vi "TDMS Advanced Asynchronous Write Speed Test.vi"() -> ()   [LabVIEW 2023]
doc: "This example demonstrates how to benchmark the streaming performance when you use the TDMS Advanced Asynchronous File I/O functions to write data to a .tdms file. This VI measures the time it takes to continuously write data from system memory to a .tdms file on the hard disk or a RAID array. This VI then calculates the average data throughput in bytes/second."
uses:
  <vilib>/Utility/tdmsutil.llb/TDMS Generate Random Data (I16).vi
panel:
  in  "Disable Buffering? (T)":bool=TRUE
  out "Bytes/second":dbl format="%#_4p"
  in  "Max Asynchronous Writes (4)":u32=4 step=1
  out "Current Number of Writes":i32
  out "Total Number of Writes":u64
  in  "Total Bytes to Write":u64=419430400
  in  "Write Block Size (bytes)":u64=4194304 step=1048576
  # "Overview: Demonstrates how to benchmark the streaming performance when you use the TDMS Advanced Asynchronous Write function to write data to a .tdms file.\nInstructions:\nRun the VI. The file is created at [LabVIEW Data]\\Example TDMS Asynchronous Speed Test Data.tdms."
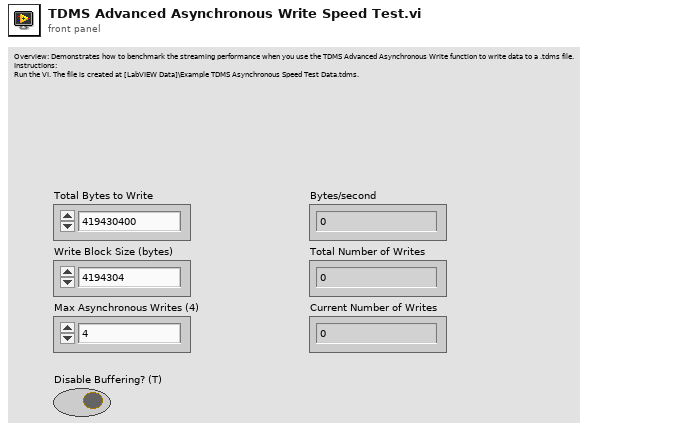
[diagram p1: front panel]
types:
  T1 = enum16{"open", "open or create", "create or replace", "create", "open (read-only)"}
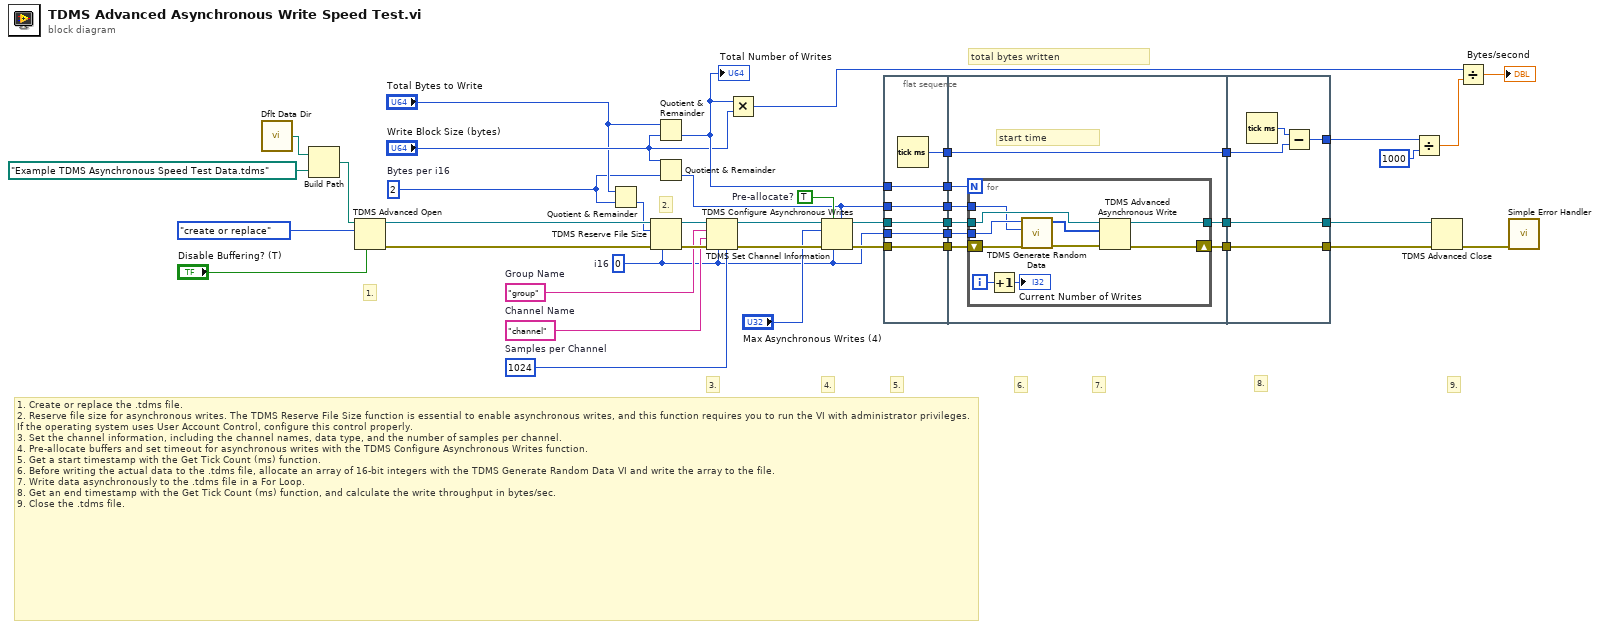
[diagram p0: block diagram]
diagram:
  w11 = TRUE  # Pre-allocate?
  w21 = "group"  # Group Name
  w19 = u64 2  # Bytes per i16
  w23 = "channel"  # Channel Name
  w13 = i16 0  # i16
  w32 = u32 1024  # Samples per Channel
  # "total bytes written"
  # "9."
  # "5."
  # "4."
  # "8."
  # "7."
  # "6."
  # "3."
  # "2."
  # "1."
  # "1. Create or replace the .tdms file.  \n2. Reserve file size for asynchronous writes. The TDMS Reserve File Size function is essential to enable asynchronous writes, and this function requires you to run the VI with administrator privileges. If the operating system uses User Account Control, configure this control properly.  \n3. Set the channel information, including the channel names, data type, and the number of samples per channel.\n4. Pre-allocate buffers and set timeout for asynchronous writes with the TDMS Configure Asynchronous Writes function.\n5. Get a start timestamp with the Get Tick Count (ms) function.\n6. Before writing the actual data to the .tdms file, allocate an array of 16-bit integers with the TDMS Generate Random Data VI and write the array to the file.\n7. Write data asynchronously to the .tdms file in a For Loop.\n8. Get an end timestamp with the Get Tick Count (ms) function, and calculate the write throughput in bytes/sec.\n9. Close the .tdms file."
  n1 = call <vilib>:"Dflt Data Dir.vi"() -> ("App:Default Data Directory"=w1:path)
  n2 = Build Path(base path=w1, name or relative path=path "Example TDMS Asynchronous Speed Test Data.tdms") -> (appended path=w2:path)
  n3 = TDMS Advanced Open(6:"Disable Buffering? (T)", 10:T1."create or replace" ("operation (0:open)"), 11:w2) -> (0:w29:errorcluster, 3:w27:refnum<k34>)  [unwired: 2 in, 1 out]
  n4 = Quotient & Remainder(x="Total Bytes to Write", y=w19) -> (floor(x/y)=w18:u64)  [unwired: 1 out]
  n5 = TDMS Reserve File Size(6:w13, 8:w29, 10:w18, 11:w27) -> (0:w28:errorcluster, 3:w26:refnum<k34>)  [unwired: 1 in]
  n6 = Quotient & Remainder(x="Total Bytes to Write", y="Write Block Size (bytes)") -> (floor(x/y)=w33:u64)  [unwired: 1 out]
  "Total Number of Writes" <- w33
  n7 = Quotient & Remainder(x="Write Block Size (bytes)", y=w19) -> (floor(x/y)=w10:u64)  [unwired: 1 out]
  n8 = TDMS Set Channel Information(4:w32, 6:w13, 8:w28, 9:w23, 10:w21, 11:w26) -> (0:w31:errorcluster, 3:w25:refnum<k34>)  [unwired: 1 in]
  n9 = Multiply(x=w33, y="Write Block Size (bytes)") -> (x*y=w6:u64)
  n10 = TDMS Configure Asynchronous Writes(5:w10, 6:w13, 7:w11, 8:w31, 10:"Max Asynchronous Writes (4)", 11:w25) -> (0:w15:errorcluster, 3:w30:refnum<k34>)  [unwired: 1 in]
  n11 = flat-sequence {
    tunnel: w30 -> [w48]
    tunnel: [w48] -> w42
    tunnel: [w47] -> w41
    tunnel: w33 -> [w46]
    tunnel: [w46] -> w40
    tunnel: [w45] -> w16
    tunnel: w15 -> [w45]
    tunnel: [w44] -> w14
    tunnel: w13 -> [w44]
    tunnel: [w43] -> w12
    tunnel: w10 -> [w43]
    tunnel: w42 -> [w56]
    tunnel: w41 -> [w55]
    tunnel: [w55] -> w39
    tunnel: [w54] -> w38
    tunnel: [w53] -> w37
    tunnel: w40 -> [w52]
    tunnel: w16 -> [w51]
    tunnel: w14 -> [w50]
    tunnel: w12 -> [w49]
    tunnel: w39 -> [w68]
    tunnel: w38 -> [w71]
    tunnel: [w71] -> w35
    tunnel: [w70] -> w34
    tunnel: w37 -> [w70]
    tunnel: [w67] -> w5
    frame #0 {
      n12 = Tick Count (ms)() -> (millisecond timer value=w47:u32)
    }
    frame #1 {
      # "start time"
      n13 = for {
        N: w52 -> [_]
        tunnel: [w63] -> w54
        shift-right: [w66] -> w53
        shift-left: w51 -> [w61]
        tunnel: w56 -> [w60]
        tunnel: w50 -> [w58]
        tunnel: w49 -> [w57]
        i -> [w65]
        n14 = Increment(x=w65) -> (x+1=→"Current Number of Writes":i32)
        n15 = call-poly <vilib>:"TDMS Generate Random Data.vi"("error in (no error)"=w61, "number of samples"=w57, "data type"=w58) -> ("error out"=w62:errorcluster, "data"=w59:i16[])  [unwired: 7 in]
        n16 = TDMS Advanced Asynchronous Write(8:w62, 10:w59, 11:w60) -> (0:w66:errorcluster, 3:w63:refnum<k34>)
      }
    }
    frame #2 {
      n17 = Tick Count (ms)() -> (millisecond timer value=w69:u32)
      n18 = Subtract(x=w69, y=w68) -> (x-y=w67:u32)
    }
  }
  n19 = Divide(x=w5, y=u32 1000) -> (x/y=w8:dbl)
  n20 = TDMS Advanced Close(8:w34, 11:w35) -> (0:w36:errorcluster)  [unwired: 2 in, 1 out]
  n21 = Divide(x=w6, y=w8) -> (x/y=→"Bytes/second":dbl)
  n22 = call <vilib>:"Simple Error Handler.vi"("error in (no error)"=w36) -> ()  [unwired: 1 in, 8 out]
